vi "Write Section Name.vi"(8 "error in (no error)":errorcluster, 10 "Section Name":string, 11 "Pages in":refnum<class "Pages.lvclass">) -> (0 "error out":errorcluster, 3 "Pages out":refnum<class "Pages.lvclass">)   [LabVIEW 2015, in "Pages.lvclass"]
uses:
  Pages.lvclass
  Pages.lvclass/Pages.ctl
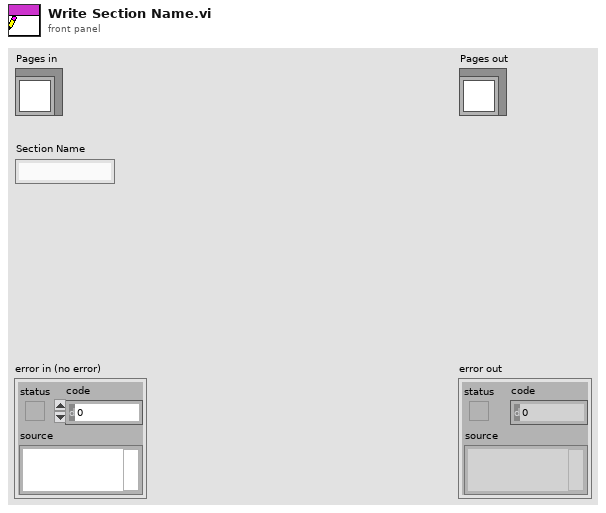
[diagram p1: front panel]
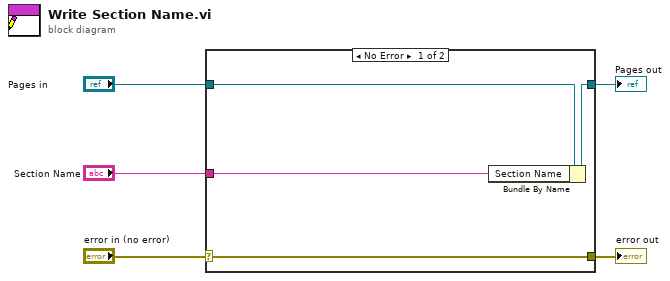
[diagram p0: block diagram]
diagram:
  n1 = case shown="No Error" "error in (no error)" {
    selector: "error in (no error)" -> [w9 w10]
    tunnel: [w9 w10] -> w4
    tunnel: [w7 w11] -> w2
    tunnel: "Pages in" -> [w8 w11]
    tunnel: "Section Name" -> [w6 _]
    frame No Error {
      n2 = Bundle By Name(cluster=w8, "Section Name"=w6) -> (w7:refnum<class "Pages.lvclass">)
    }
    frame Error {
    }
  }
  "error out" <- w4
  "Pages out" <- w2
